vi "FlexDDS-NG_DCP_Reset.vi"(9 "full reset (yes)":bool=TRUE, 10 "Channels":T1(ring)=enum."Both channels", 11 "initial instruction string":string) -> (3 "appended instruction string":string="dds reset\r")   [LabVIEW 2010]
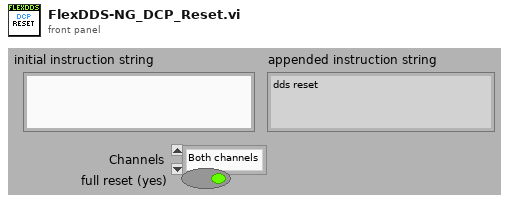
[diagram p1: front panel]
types:
  T1 = enum32{"Channel 0", "Channel 1", "Both channels"}
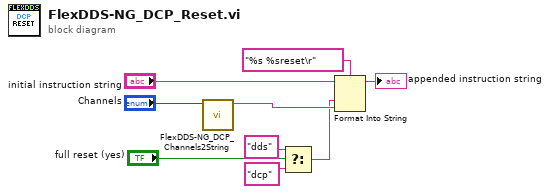
[diagram p0: block diagram]
diagram:
  n1 = call "FlexDDS-NG_DCP_Channels2String.vi"("Channels"="Channels") -> ("channels string"=w5:string)  [unwired: 10 in]
  n2 = Select(t="dds" ("format string"), s="full reset (yes)", f="dcp" ("format string")) -> (s? t:f=w3:string)
  n3 = Format Into String(format string="%s %sreset\r", initial string="initial instruction string", w3, w5) -> (resulting string=→"appended instruction string":string)  [unwired: 1 in, 1 out]
